vi "mupEval.vi"(8 "error in (no error)":errorcluster, 11 "hParser in":u64) -> (0 "error out":errorcluster, 2 "result":dbl, 3 "hParser out":u64)   [LabVIEW 2015, in "muParser.lvlib"]
uses:
  muParser.lvlib
  <vilib>/Utility/error.llb/Error Cluster From Error Code.vi
  muparser.dll
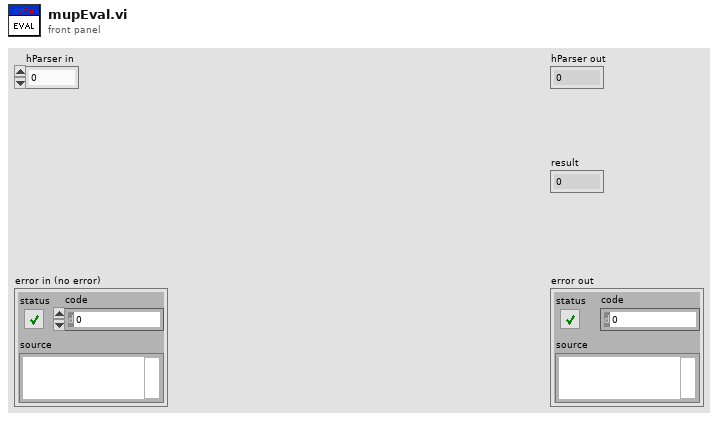
[diagram p1: front panel]
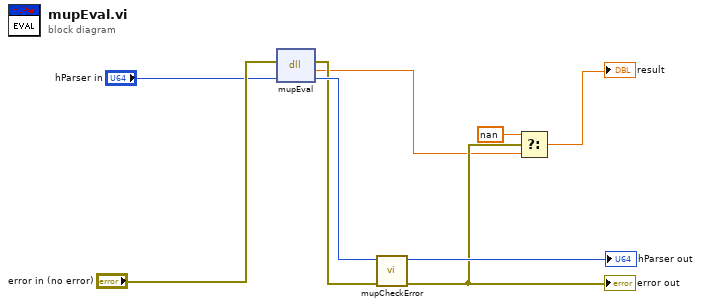
[diagram p0: block diagram]
diagram:
  n1 = dll-call lib="C:/Users/porter/Documents/GitHub/LV-muParser/muparser.dll" fn="mupEval"(error in="error in (no error)", "hParser"="hParser in") -> (error out=w8:errorcluster, "return type"=w3:dbl, "hParser"=w9:u64)  [unwired: 2 in, 1 out]
  n2 = call "mupCheckError.vi"("error in (no error)"=w8, "hParser in"=w9) -> ("error out"=w4:errorcluster, "hParser out"=→"hParser out":u64)  [unwired: 8 in]
  "error out" <- w4
  n3 = Select(t=nan, s=w4, f=w3) -> (s? t:f=→"result":dbl)
